vi "AWG Write Multiple Scripts.vi"(8 "error in":errorcluster, 10 "Scripts":string[](array[string])=["script myScript0\n      Generate TRise\n      Generate THi\n      Generate TFall\n      Generate WaitLo\n      Generate BRise\n      Generate BHi\n      Generate BFall\n      Generate WaitLo\nend script", "script myScript1\n      Wait until scriptTrigger0\n      Generate TRise\n      Generate THi\n      Generate TFall\n      Generate WaitLo\n      Generate BRise\n      Generate BHi\n      Generate BFall\n      Generate WaitLo\nend script"], 11 "Semiconductor Module Context":T1) -> (0 "error out":errorcluster)   [LabVIEW 2013]
uses:
  <vilib>/NI_TestStand_SemiconductorModule/NI_TestStand_Semiconductor_Module.lvlibp/PinMap/General/SemiconductorModuleContext.ctl
  <vilib>/NI_TestStand_SemiconductorModule/NI_TestStand_Semiconductor_Module.lvlibp
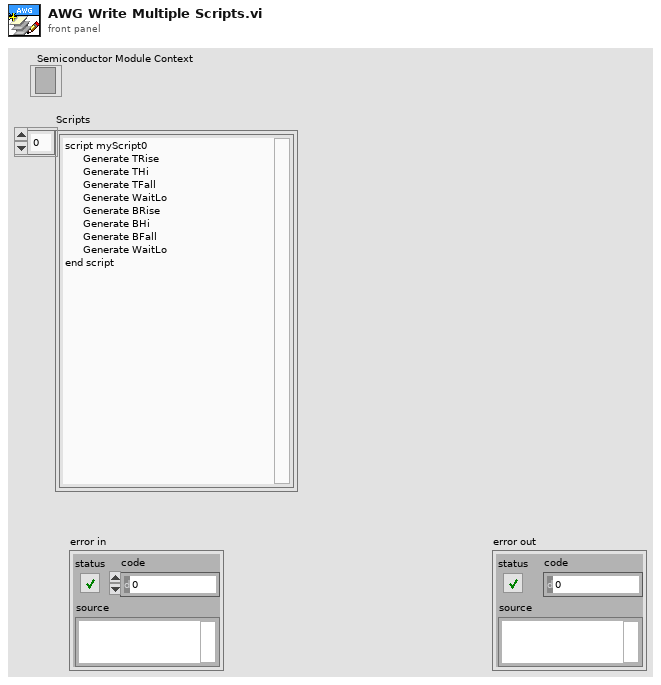
[diagram p1: front panel]
types:
  T1 = typedef "NI_TestStand_Semiconductor_Module.lvlibp/SemiconductorModuleContext.ctl" = refnum<k7>
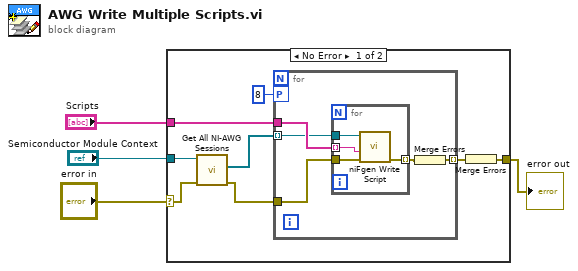
[diagram p0: block diagram]
diagram:
  n1 = case shown="No Error" "error in" {
    selector: "error in" -> [w5 w22]
    tunnel: "Scripts" -> [w12 _]
    tunnel: [w10 w22] -> w3
    tunnel: "Semiconductor Module Context" -> [w6 _]
    frame No Error {
      n2 = call "Get All NI-AWG Sessions.vi"("error in (no error)"=w5, "Semiconductor Module Context"=w6) -> ("error out"=w7:errorcluster, "Instrument Sessions"=w8:refnum<k15>[])  [unwired: 7 in, 1 out]
      n3 = for {
        tunnel: w12 -> [w17]
        tunnel: w7 -> [w16]
        tunnel: [w14] -> w11 mode=indexing
        workers-P: 8 -> [_]
        tunnel: w8 -> [w13] mode=indexing
        n4 = for {
          tunnel: w13 -> [w21]
          tunnel: w16 -> [w20]
          tunnel: w17 -> [w19] mode=indexing
          tunnel: [w18] -> w15 mode=indexing
          n5 = call <instrlib>:"niFgen Write Script.vi"("error in (no error)"=w20, "Script"=w19, "Instrument Handle"=w21) -> ("error out"=w18:errorcluster)  [unwired: 7 in, 1 out]
        }
        n6 = Merge Errors(w15) -> (w14:errorcluster)
      }
      n7 = Merge Errors(w11) -> (w10:errorcluster)
    }
    frame Error {
    }
  }
  "error out" <- w3
